vi "Convert Read ERD List to Message.vi"(0 "GEA Inputs":T1 {"Destination" format="%.0x"; "Source" format="%.0x"}, 7 "Read ERD List":T3[](array[typedef]) {"ERD Number" format="%.0x"}, 11 "Error In":errorcluster) -> (4 "GEA Message":T2 {"Command" format="%02x"; "Destination" format="%02x"; "Source" format="%02x"}, 15 "Error Out":errorcluster)   [LabVIEW 2014, in "GEA2_Toolkit.lvlib"]
doc: "This vi uses the Source / Destination from the GEA input and the ERD list to format a single GEA2 message to read the list of ERDs."
uses:
  library/GEA2_Toolkit.lvlib
  type defs/ERD Read Data In.ctl
  type defs/Data In.ctl
  type defs/Source_Destination.ctl
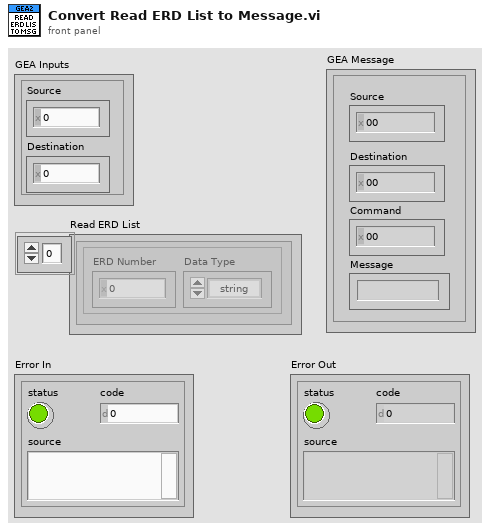
[diagram p1: front panel]
types:
  T1 = typedef "GEA2_Toolkit.lvlib/Source_Destination.ctl" = cluster{"Source":u8, "Destination":u8}
  T2 = typedef "GEA2_Toolkit.lvlib/Data In.ctl" = cluster{"Source":u8, "Destination":u8, "Command":u8, "Message":string}
  T3 = typedef "GEA2_Toolkit.lvlib/ERD Read Data In.ctl" = cluster{"ERD Number":u16, "Data Type":enum16{"string", "boolean", "uint8_t", "uint16_t", "uint32_t", "uint64_t"}}
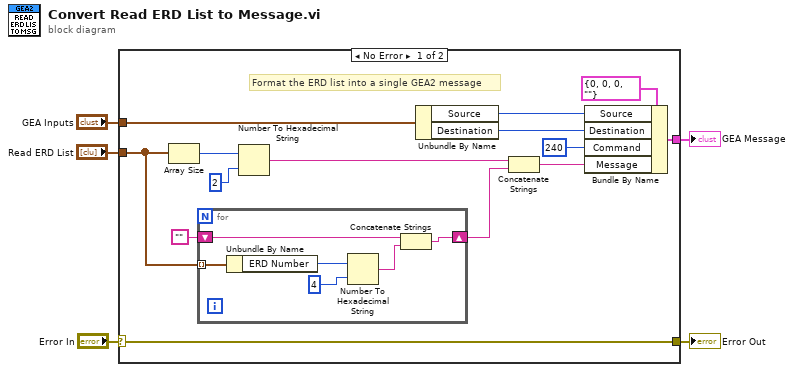
[diagram p0: block diagram]
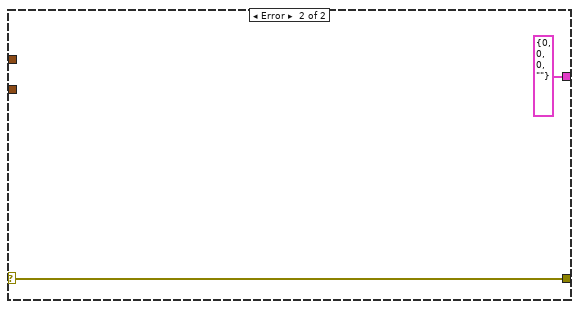
[diagram p2: hidden frame]
diagram:
  n1 = case shown="No Error" "Error In" {
    selector: "Error In" -> [w6 w26]
    tunnel: "Read ERD List" -> [w16 _]
    tunnel: "GEA Inputs" -> [w12 _]
    tunnel: [w7 T2 {"Source"=0, "Destination"=0, "Command"=0, "Message"=""} ("GEA Message")] -> w3
    tunnel: [w6 w26] -> w1
    frame No Error {
      # "Format the ERD list into a single GEA2 message"
      n2 = Array Size(array=w16) -> (size(s)=w18:i32)
      n3 = for {
        tunnel: w16 -> [w25] mode=indexing
        shift-right: [w20] -> w14
        shift-left: "" -> [w22]
        n4 = Unbundle By Name(w25) -> ("ERD Number"=w24:u16)
        n5 = Number To Hexadecimal String(1:i16 4 ("width (-)"), 2:w24) -> (0:w21:string)
        n6 = Concatenate Strings(w22, w21) -> (w20:string)
      }
      n7 = Number To Hexadecimal String(1:i16 2 ("width (-)"), 2:w18) -> (0:w17:string)
      n8 = Unbundle By Name(w12) -> ("Source"=w11:u8, "Destination"=w10:u8)
      n9 = Concatenate Strings(w17, w14) -> (w8:string)
      n10 = Bundle By Name(cluster=T2 {"Source"=0, "Destination"=0, "Command"=0, "Message"=""} ("GEA Message"), "Source"=w11, "Destination"=w10, "Command"=u8 240, "Message"=w8) -> (w7:T2)
    }
    frame Error {
    }
  }
  "GEA Message" <- w3
  "Error Out" <- w1
